vi "Perform Bode Analysis.vi"(5 "Y Maximum (60)":dbl=60.0, 7 "Y Minimum (-60)":dbl=-60.0, 8 "error in (no error)":errorcluster, 9 "Frequency Stop (20000000: 20000000)":i32(ring)=20000000 items=["100"=100, "1000"=1000, "10000"=10000, "100000"=100000, "1000000"=1000000, "10000000"=10000000, "20000000"=20000000], 10 "Frequency Start (100: 100)":i32(ring)=100 items=["20"=20, "100"=100, "1000"=1000, "10000"=10000, "100000"=100000, "1000000"=1000000, " 10000000"=10000000], 11 "VISA resource name":refnum<visa-resource-name>) -> (0 "error out":errorcluster, 3 "VISA resource name out":refnum<visa-resource-name>)   [LabVIEW 2023, in "Keysight-DSQx3014T.lvlib"]
doc: "Performs the control loop response (Bode) analysis to help you determine the margin of a control loop. \n\nA Bode plot measurement plots gain (A) in units of dB as a function of frequency.\nThis control loop response analysis requires an input sine wave (from the oscilloscope's waveform generator, Vi) be swept from a low to a high frequency\nwhile measuring Vi and Vo RMS voltages at each step frequency, using two\nchannels of the oscilloscope. Gain (A) at each step frequency is computed as\n20Log(Vo/Vi) and plotted using a math function waveform.\n\nIt takes some time for the frequency sweep analysis to complete. You can query bit\n0 of the Standard Event Status Register (*ESR?) to find out when the analysis is complete."
uses:
  Keysight-DSQx3014T.lvlib
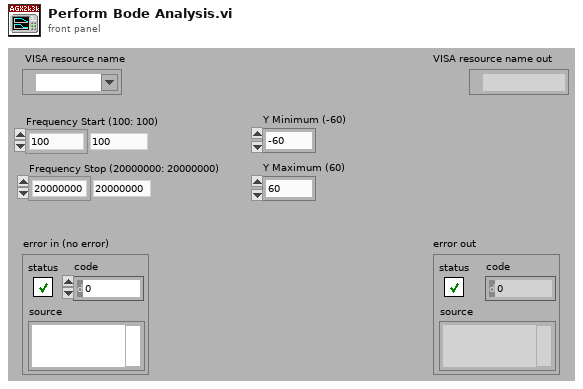
[diagram p1: front panel]
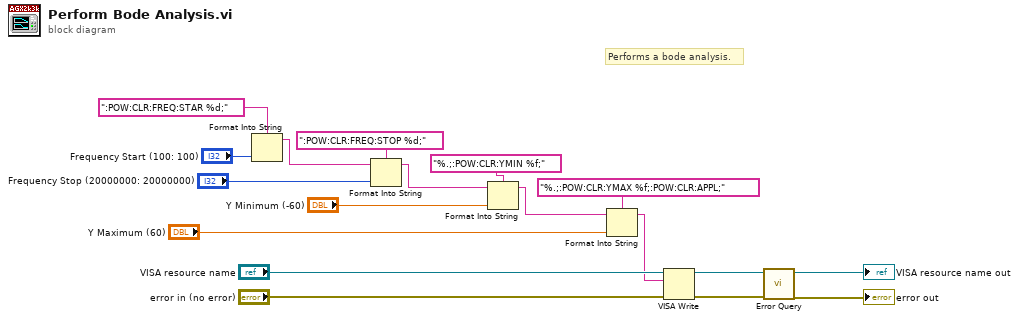
[diagram p0: block diagram]
diagram:
  # "Performs a bode analysis."
  n1 = Format Into String(format string=":POW:CLR:FREQ:STAR %d;", "Frequency Start (100: 100)") -> (resulting string=w8:string)  [unwired: 2 in, 1 out]
  n2 = Format Into String(format string=":POW:CLR:FREQ:STOP %d;", initial string=w8, "Frequency Stop (20000000: 20000000)") -> (resulting string=w6:string)  [unwired: 1 in, 1 out]
  n3 = Format Into String(format string="%.;:POW:CLR:YMIN %f;", initial string=w6, "Y Minimum (-60)") -> (resulting string=w3:string)  [unwired: 1 in, 1 out]
  n4 = Format Into String(format string="%.;:POW:CLR:YMAX %f;:POW:CLR:APPL;", initial string=w3, "Y Maximum (60)") -> (resulting string=w1:string)  [unwired: 1 in, 1 out]
  n5 = VISA Write(VISA resource name="VISA resource name", write buffer=w1, error in (no error)="error in (no error)") -> (VISA resource name out=w16:refnum<visa-resource-name>, error out=w15:errorcluster)  [unwired: 1 out]
  n6 = call "Error Query.vi"("error in (no error)"=w15, "VISA resource name"=w16) -> ("error out"=→"error out":errorcluster, "VISA resource name out"=→"VISA resource name out":refnum<visa-resource-name>)  [unwired: 8 out]
